vi "Move Lift.vi"() -> ()   [LabVIEW 2014]
panel:
  in  "Encoder B":dbl
  in  "Encoder A":dbl
  in  "Move Down":dbl
  in  "Move Up":dbl
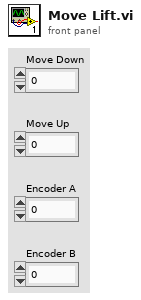
[diagram p1: front panel]
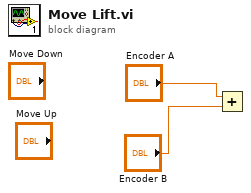
[diagram p0: block diagram]
diagram:
  n1 = Add(x="Encoder A", y="Encoder B") -> ()  [unwired: 1 out]
